vi "Autonomous Independent.vi"   [LabVIEW 2011]
doc: "This VI is called when autonomous begins, and will automatically be terminated when autonomous ends. You can carry out timed or sensor driven robot movement independently without needing to return to the caller."
uses:
  Robot Global Data.vi
  <vilib>/Rock Robotics/WPI/Solenoid/Deprecated/WPI_SolenoidSetBool.vi
types:
  T1 = typedef "WPI_JoystickDevRef.ctl" = cluster{"Device":T2}
  T2 = typedef "WPI_JoystickDeviceEnum.ctl" = enum16{"USB 1", "USB 2", "USB 3", "USB 4", "Kinect 1", "Kinect 2"}
  T3 = cluster{"axis 1 (x)":dbl, "axis 2 (y)":dbl, "axis 3 (throttle)":dbl, "axis 4":dbl, "axis 5":dbl, "axis 6":dbl}
  T4 = enum16{"Tip Bridge", "No Bridge", "Kinect Bridge"}
  T5 = typedef "WPI_SolenoidDevRef.ctl" = cluster{"DevStatus":errorcluster, "Solenoid Module":T6, "Forward Solenoid Channel":T7, "Reverse Solenoid Channel":T7}
  T6 = typedef "FPGA_TypedefSolenoidModule.ctl" = enum16{"Solenoid Module 1", "Solenoid Module 2"}
  T7 = typedef "WPI_SolenoidChannel.ctl" = enum8{"Solenoid 1", "Solenoid 2", "Solenoid 3", "Solenoid 4", "Solenoid 5", "Solenoid 6", "Solenoid 7", "Solenoid 8", "Invalid"}
  T8 = typedef "UDP Dashboard Packet TypeDef.ctl" = cluster{"Distance":dbl, "Shooter Control":cluster{"Manual Enabled":bool, "Manual Distance":dbl, "Power Constant":dbl, "RPM Constant":dbl, "Layup Distance":dbl, "RPM Range":cluster{"Max Percentage":dbl, "Min Percentage":dbl}, "Dt In":dbl}, "Tracking Setpoint":dbl, "Shooter PID gains":cluster{"proportional gain (Kc)":dbl, "integral time (Ti, min)":dbl, "derivative time (Td, min)":dbl}, "Tracking PID gains":cluster{"proportional gain (Kc)":dbl, "integral time (Ti, min)":dbl, "derivative time (Td, min)":dbl}, "Shooter PID gains 2":cluster{"proportional gain (Kc)":dbl, "integral time (Ti, min)":dbl, "derivative time (Td, min)":dbl}, "Tracking Tolerance":dbl, "Tracking Limit":dbl, "Autonomous Ball Collection / Shoot Period":dbl}
  T9 = typedef "WPI_GyroDevRef.ctl" = cluster{"DevStatus":errorcluster, "Analog Module":T10, "Analog Channel":T11, "Offset":dbl, "Gain (VoltsPerDegree/Second)":dbl}
  T10 = typedef "FPGA_TypedefAnalogModule.ctl" = enum16{"Analog Module 1", "Analog Module 2"}
  T11 = typedef "FPGA_AIChannel.ctl" = enum8{"AI 1", "AI 2", "AI 3", "AI 4", "AI 5", "AI 6", "AI 7", "AI 8", "Invalid"}
  T12 = typedef "WPI_RobotDriveDevRef.ctl" = cluster{"DevStatus":errorcluster, "Motors[]":T13[], "Square Inputs":bool, "Max Output":dbl, "Isochronous":bool}
  T13 = typedef "WPI_MotorControlDeviceRef.ctl" = cluster{"DeviceStatus":errorcluster, "Type":enum16{"PWM", "CAN"}, "PWM":cluster{"Digital Module":T14, "PWM Channel":T15, "DeadBand":T16}, "CAN":cluster{"Device Number":u8, "Control Mode":T17, "Semaphore":T18, "Max Vout":dbl}, "Invert":bool, "TransformRef":T19, "InvTransformRef":T19}
  T14 = typedef "FPGA_TypedefDigitalModule.ctl" = enum16{"Digital Module 1", "Digital Module 2"}
  T15 = typedef "FPGA_DIOPWMChannel.ctl" = enum8{"PWM 1", "PWM 2", "PWM 3", "PWM 4", "PWM 5", "PWM 6", "PWM 7", "PWM 8", "PWM 9", "PWM 10", "Invalid"}
  T16 = typedef "WPI_PWMDeadband.ctl" = cluster{"Name":string, "maxPositivePwm":i32, "minPositivePwm":i32, "centerPwm":i32, "maxNegativePwm":i32, "minNegativePwm":i32, "angularRange":u16}
  T17 = typedef "WPI_CANJaguar_ControlMode.ctl" = enum8{"Percent VBus", "Current", "Speed", "Position", "Voltage"}
  T18 = typedef "Semaphore RefNum" = refnum<k1>
  T19 = typedef "WPI_PWMTransform_ConPane.ctl" = refnum<vi>
  T20 = cluster{"Shooter Warmup":bool, "Shooter Allow Fire":bool}
  T21 = typedef "WPI_EncoderDevRef.ctl" = cluster{"DevStatus":errorcluster, "EncoderIndex":T22, "CounterIndex":T23, "DistancePerCount":dbl, "Decoding Type":T24}
  T22 = typedef "FPGA_EncoderIdx.ctl" = enum8{"Enc 0", "Enc 1", "Enc 2", "Enc 3", "Invalid"}
  T23 = typedef "FPGA_CounterCtrSystemIndex.ctl" = enum8{"Ctr 0", "Ctr 1", "Ctr 2", "Ctr 3", "Ctr 4", "Ctr 5", "Ctr 6", "Ctr 7", "Invalid"}
  T24 = typedef "WPI_EncoderType.ctl" = enum16{"1x", "2x", "4x"}
  T25 = typedef "WPI_DigitalInputDevRef.ctl" = cluster{"DevStatus":errorcluster, "DIO Channel":T26, "Digital Module":T14}
  T26 = typedef "FPGA_DIOChannel.ctl" = enum8{"DIO 1", "DIO 2", "DIO 3", "DIO 4", "DIO 5", "DIO 6", "DIO 7", "DIO 8", "DIO 9", "DIO 10", "DIO 11", "DIO 12", "DIO 13", "DIO 14", "Invalid"}
  T27 = typedef "WPI_JoystickButtonState.ctl" = cluster{"Button 1":bool, "Button 2":bool, "Button 3":bool, "Button 4":bool, "Button 5":bool, "Button 6":bool, "Button 7":bool, "Button 8":bool, "Button 9":bool, "Button 10":bool, "Button 11":bool, "Button 12":bool}
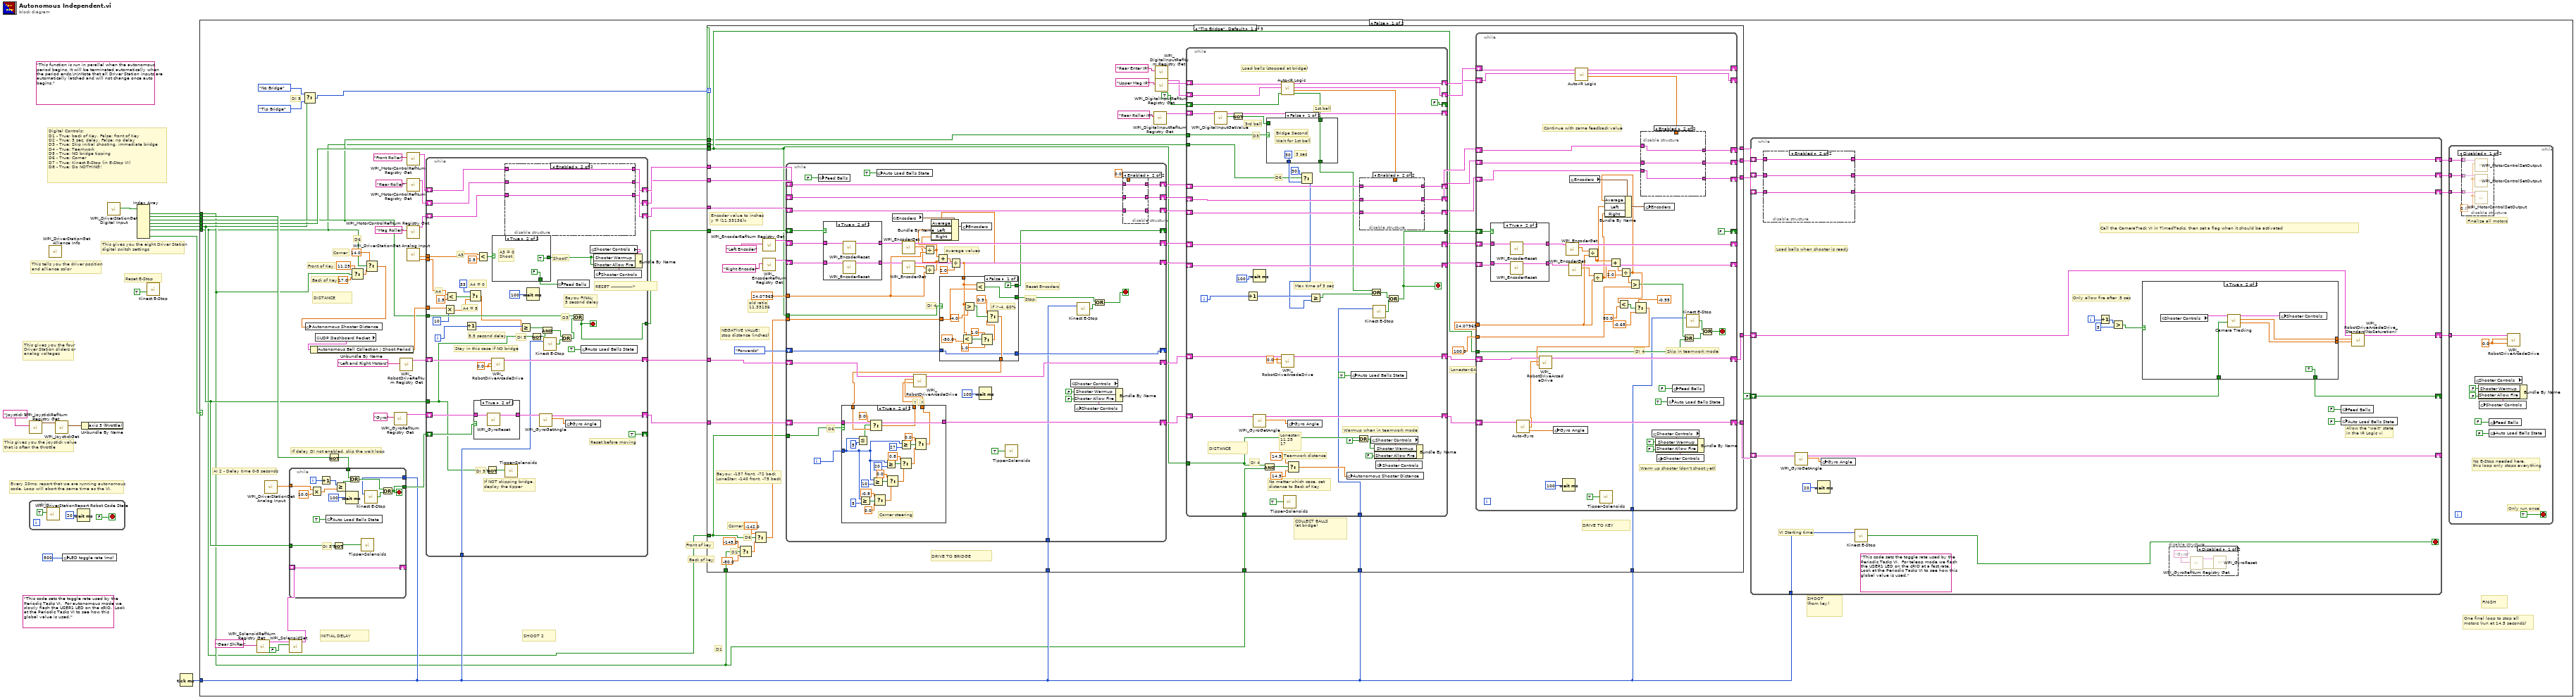
[diagram p0: block diagram]
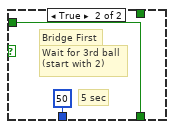
[diagram p3: hidden frame]
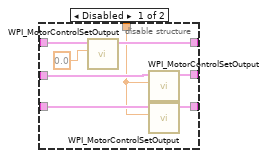
[diagram p4: hidden frame]
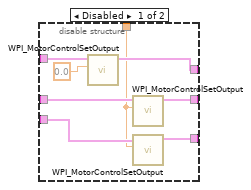
[diagram p5: hidden frame]
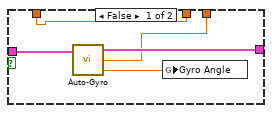
[diagram p7: hidden frame]
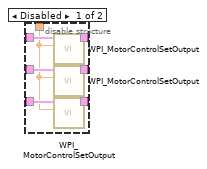
[diagram p8: hidden frame]
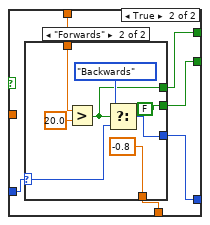
[diagram p9: hidden frame]
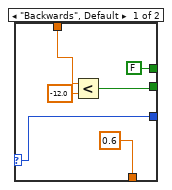
[diagram p10: hidden frame]
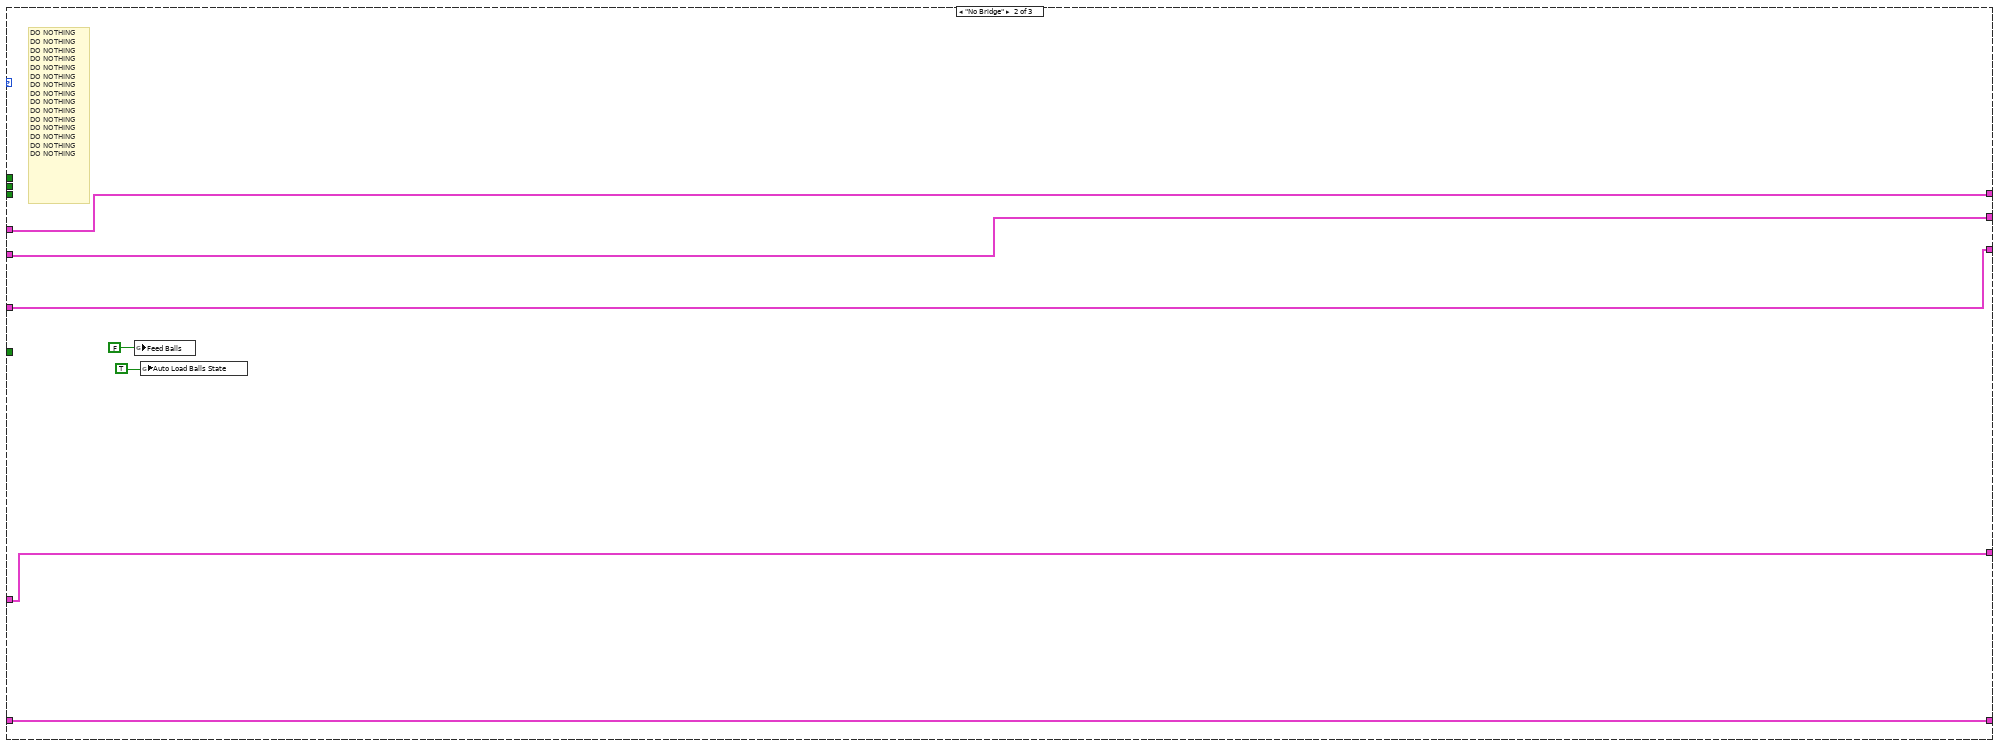
[diagram p12: hidden frame]
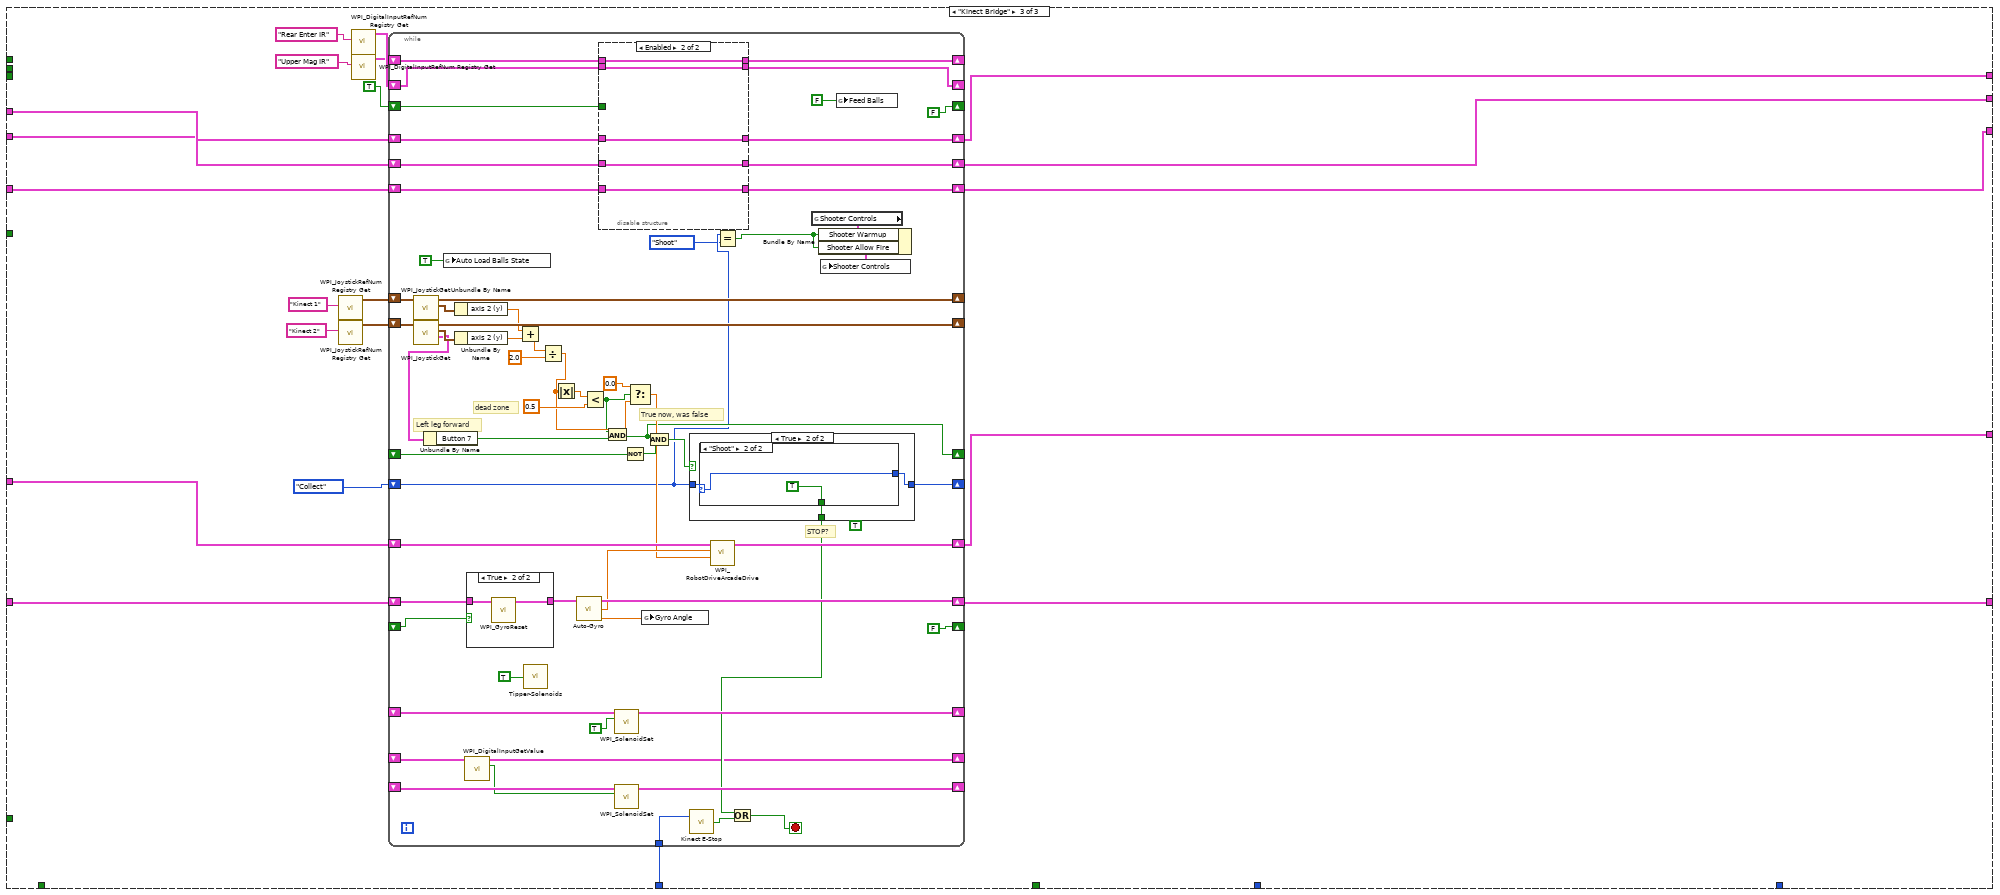
[diagram p13: hidden frame]
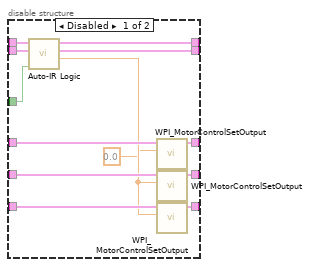
[diagram p14: hidden frame]
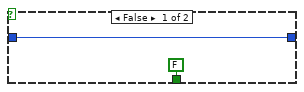
[diagram p15: hidden frame]
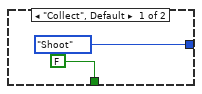
[diagram p16: hidden frame]
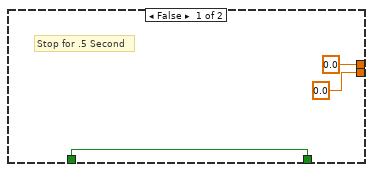
[diagram p18: hidden frame]
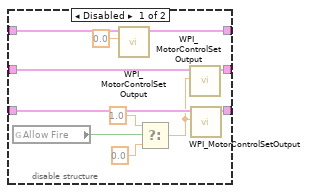
[diagram p20: hidden frame]
diagram:
  (unwired) "This code sets the toggle rate used by the Periodic Tasks VI.  For autonomous mode we slowly flash the USER1 LED on the cRIO.  Look at the Periodic Tasks VI to see how this global value is used."
  (unwired) "This function is run in parallel when the autonomous period begins. It will be terminated automatically when the period ends.\n\nNote that all Driver Station inputs are automatically latched and will not change once auto begins."
  # "Reset E-Stop"
  # "Digital Controls:\nD1 - True: back of Key, False: front of Key\nD2 - True: 3 sec. delay, False: no delay\nD3 - True: Skip initial shooting, immediate bridge\nD4 - True: Teamwork\nD5 - True: NO bridge tipping\nD6 - True: Corner\nD7 - True: Kinect E-Stop (in E-Stop VI)\nD8 - True: Do NOTHING!"
  # "Every 20ms, report that we are running autonomous\ncode. Loop will abort the same time as the VI."
  # "This gives you the joystick value\nthat is often the throttle"
  # "This tells you the driver position\nand alliance color"
  # "This gives you the eight Driver Station\ndigital switch settings"
  # "This gives you the four\nDriver Station sliders or\nanalog voltages"
  n1 = call <vilib>:"WPI_JoystickRefNum Registry Get.vi"("refnum name"="Joystick 1") -> ("JoystickDevRef"=w11:T1)  [unwired: 1 in, 9 out]
  n2 = while {
    stop <- FALSE stop-if-true
    n3 = call <vilib>:"WPI_DriverStationReport Robot Code State.vi"("Autonomous"=TRUE) -> ()  [unwired: 10 in, 1 out]
    n4 = Wait (ms)(milliseconds to wait=u32 20) -> ()  [unwired: 1 out]
  }
  n5 = call <vilib>:"WPI_DriverStationGet Alliance Info.vi"() -> ()  [unwired: 12 out]
  n6 = call <vilib>:"WPI_JoystickGet.vi"("JoystickDevRef"=w11) -> ("Axes"=w12:T3)  [unwired: 1 in, 5 out]
  n7 = global write "Robot Global Data.vi" "LED toggle rate (ms)"(u32 500 ("LED ms toggle rate")) -> ()
  n8 = Unbundle By Name(w12) -> ()  [unwired: 1 out]
  n9 = call <vilib>:"WPI_DriverStationGet Digital Input.vi"() -> ("Driver Station Digital Input (1-8)"=w14:bool[])  [unwired: 11 out]
  n10 = Index Array(array=w14) -> (element #1=w7:bool, element #2=w9:bool, element #3=w1:bool, element #4=w8:bool, element #5=w5:bool, element #6=w2:bool, element #8=w6:bool)  [unwired: 8 in, 1 out]
  n11 = call "Kinect E-Stop.vi"("Reset"=TRUE) -> ()  [unwired: 1 in, 1 out]
  n12 = Tick Count (ms)() -> (millisecond timer value=w4:u32)
  n13 = case shown="False" w6 {
    tunnel: w9 -> [w45 _]
    tunnel: w8 -> [w43 _]
    tunnel: w7 -> [w24 _]
    tunnel: w5 -> [w26 _]
    tunnel: w4 -> [w36 _]
    tunnel: w2 -> [w18 _]
    tunnel: w1 -> [w27 _]
    frame False {
      # "Back of key"
      # "Front of key"
      # "Corner"
      # "D6"
      # "Back of Key"
      # "Front of Key"
      # "RESET --------------->"
      # "FINISH"
      # "SHOOT\n(from key)"
      # "AI 2 - Delay time 0-5 seconds"
      # "SHOOT 2"
      # "INITIAL DELAY"
      # "If delay DI not enabled, skip the wait loop"
      # "One final loop to stop all\nmotors (run at 14.5 seconds)"
      # "DI 5"
      # "DISTANCE"
      # "D1"
      n14 = call <vilib>:"WPI_SolenoidRefNum Registry Get.vi"("refnum name"="Gear Shifter") -> ("SolenoidDevRef"=w34:T5)  [unwired: 9 in, 1 out]
      n15 = call <vilib>:"WPI_DriverStationGet Analog Input.vi"() -> ("Analog 2 (V)"=w44:dbl)  [unwired: 11 out]
      n16 = call-poly <vilib>:"WPI_SolenoidSet.vi"("Value"=FALSE, "SolenoidDevRef"=w34) -> ("SolenoidDevRef"=w33:T5)  [unwired: 8 in, 1 out]
      n17 = Select(t=T4."No Bridge", s=w26, f=T4."Tip Bridge") -> (s? t:f=w25:T4)
      n18 = global read "Robot Global Data.vi" "UDP Dashboard Packet"() -> (w29:T8)
      n19 = Unbundle By Name(w29) -> ("Autonomous Ball Collection / Shoot Period"=w28:dbl)
      n20 = Not(x=w45) -> (.not. x?=w46:bool)
      n21 = while {
        tunnel: [w539] -> w47
        tunnel: w46 -> [w545]
        tunnel: w44 -> [w542]
        shift-right: [w537] -> _
        shift-left: w33 -> [w537]
        tunnel: w36 -> [w538]
        tunnel: w26 -> [w535]
        i -> [w547]
        stop <- w539 stop-if-true
        # "DI 5"
        n22 = Multiply(x=w542, y=10.0) -> (x*y=w544:dbl)
        n23 = Increment(x=w547) -> (x+1=w548:i32)
        n24 = global write "Robot Global Data.vi" "Auto Load Balls State"(TRUE ("Feed Balls")) -> ()
        n25 = Not(x=w535) -> (.not. x?=w536:bool)
        n26 = Greater Or Equal?(x=w548, y=w544) -> (x >= y?=w549:bool)
        n27 = Wait (ms)(milliseconds to wait=u32 100) -> ()  [unwired: 1 out]
        n28 = Or(x=w545, y=w549) -> (x .or. y?=w540:bool)
        n29 = call "Tipper-Solenoids.vi"("Deploy Tipper"=w536) -> ()  [unwired: 1 out]
        n30 = call "Kinect E-Stop.vi"("Start Time"=w538) -> ("Stop"=w541:bool)  [unwired: 1 in]
        n31 = Or(x=w540, y=w541) -> (x .or. y?=w539:bool)
      }
      n32 = Select(t=11.25 ("X axis value"), s=w24, f=17.0 ("X axis value")) -> (s? t:f=w21:dbl)
      n33 = Select(t=14.0 ("X axis value"), s=w18, f=w21) -> (s? t:f=w20:dbl)
      n34 = global write "Robot Global Data.vi" "Autonomous Shooter Distance"(w20) -> ()
      n35 = call <vilib>:"WPI_GyroRefNum Registry Get.vi"("refnum name"="Gyro") -> ("GyroDevRef"=w50:T9)  [unwired: 9 in, 1 out]
      n36 = call <vilib>:"WPI_RobotDriveRefNum Registry Get.vi"("refnum name"="Left and Right Motors") -> ("RobotDriveDevRef"=w59:T12)  [unwired: 9 in, 1 out]
      n37 = call <vilib>:"WPI_MotorControlRefNum Registry Get.vi"("refnum name"="Front Roller") -> ("MotorControlDevRef"=w65:T13)  [unwired: 9 in, 1 out]
      n38 = call <vilib>:"WPI_MotorControlRefNum Registry Get.vi"("refnum name"="Rear Roller") -> ("MotorControlDevRef"=w64:T13)  [unwired: 9 in, 1 out]
      n39 = call <vilib>:"WPI_MotorControlRefNum Registry Get.vi"("refnum name"="Mag Roller") -> ("MotorControlDevRef"=w68:T13)  [unwired: 9 in, 1 out]
      n40 = call <vilib>:"WPI_DriverStationGet Analog Input.vi"() -> ("Analog 4 (V)"=w30:dbl, "Analog 3 (V)"=w31:dbl)  [unwired: 8 in, 2 out]
      n41 = while {
        tunnel: [w621] -> w57
        shift-right: [w639] -> w63
        shift-left: w65 -> [w641]
        shift-right: [w638] -> w62
        shift-left: w64 -> [w640]
        shift-right: [w637] -> w61
        shift-left: w68 -> [w642]
        shift-right: [w634] -> w58
        shift-left: w59 -> [w635]
        shift-right: [w626] -> w49
        shift-left: w50 -> [w631]
        shift-right: [TRUE ("Shooter Enabled")] -> _
        shift-left: w47 -> [w630]
        tunnel: w36 -> [w624]
        tunnel: w26 -> [w600]
        tunnel: w27 -> [w622]
        tunnel: w31 -> [w608]
        tunnel: w30 -> [w606]
        tunnel: w28 -> [w611]
        i -> [w633]
        stop <- w621 stop-if-true
        w636 = 0.0 ("X axis value")
        # "Stay in this case if NO bridge"
        # "DI 5"
        # "A4"
        # "A3"
        # "A4 = 0"
        # "A4 = 5"
        # "Shoot?"
        # "Reset before moving"
        # "D3"
        # "If NOT skipping bridge,\ndeploy the tipper"
        # "DI 5"
        # "Bayou FINAL:\n5 second delay"
        # "5.5 second delay"
        n42 = Multiply(x=w611, y=u32 10) -> (x*y=w612:dbl)
        n43 = Less?(x=w606, y=2.5) -> (x < y?=w605:bool)
        n44 = Increment(x=w633) -> (x+1=w632:i32)
        n45 = Select(t=u32 33 ("y"), s=w605, f=w612) -> (s? t:f=w614:dbl)
        n46 = case shown="True" w630 {
          tunnel: w631 -> [w662 w664]
          tunnel: [w662 w663] -> w627
          frame False {
          }
          frame True {
            n47 = call <vilib>:"WPI_GyroReset.vi"("GyroDevRef"=w664) -> ("GyroDevRef"=w663:T9)  [unwired: 9 in, 1 out]
          }
        }
        n48 = Less?(x=w608, y=2.5) -> (x < y?=w607:bool)
        n49 = Not(x=w600) -> (.not. x?=w623:bool)
        n50 = call-poly <vilib>:"WPI_RobotDriveArcadeDrive.vi"("Y axis value"=w636, "X axis value"=w636, "RobotDriveDevRef"=w635) -> ("RobotDriveDevRef"=w634:T12)  [unwired: 7 in, 1 out]
        n51 = case shown="True" w607 {
          tunnel: [FALSE ("Shooter Enabled") TRUE ("Shooter Enabled")] -> w619
          tunnel: [TRUE ("Shooter Enabled") FALSE ("Shooter Enabled")] -> w616
          frame False {
            # "A3 = 5\nFeed Balls Out"
          }
          frame True {
            # "A3 = 0\nShoot"
          }
        }
        n52 = disable-structure shown="Enabled" {
          disable-tunnel: w642 -> [w658 w659]
          disable-tunnel: w641 -> [w657 w661]
          disable-tunnel: w640 -> [w656 w660]
          disable-tunnel: [w654 w661] -> w639
          disable-tunnel: [w653 w660] -> w638
          disable-tunnel: [w652 w659] -> w637
          frame Disabled {
            # "Load balls when shooter is ready"
            n53 = global read "Robot Global Data.vi" "Allow Fire"() -> (w651:bool)
            n54 = Select(t=1.0 ("Output"), s=w651, f=0.0 ("Output")) -> (s? t:f=w648:dbl)
            n55 = call <vilib>:"WPI_MotorControlSetOutput.vi"("Output"=0.0, "MotorControlDevRef"=w657) -> ("MotorControlDevRef"=w654:T13)  [unwired: 8 in, 1 out]
            n56 = call <vilib>:"WPI_MotorControlSetOutput.vi"("Output"=w648, "MotorControlDevRef"=w656) -> ("MotorControlDevRef"=w653:T13)  [unwired: 8 in, 1 out]
            n57 = call <vilib>:"WPI_MotorControlSetOutput.vi"("Output"=w648, "MotorControlDevRef"=w658) -> ("MotorControlDevRef"=w652:T13)  [unwired: 8 in, 1 out]
          }
          frame Enabled {
          }
        }
        n58 = call "Tipper-Solenoids.vi"("Deploy Tipper"=w623) -> ()  [unwired: 1 out]
        n59 = Greater Or Equal?(x=w632, y=w614) -> (x >= y?=w602:bool)
        n60 = Wait (ms)(milliseconds to wait=u32 100) -> ()  [unwired: 1 out]
        n61 = Not(x=w600) -> (.not. x?=w601:bool)
        n62 = call <vilib>:"WPI_GyroGetAngle.vi"("GyroDevRef"=w627) -> ("Angle"=w628:dbl, "GyroDevRef"=w626:T9)  [unwired: 7 in, 2 out]
        n63 = And(x=w602, y=w601) -> (x .and. y?=w603:bool)
        n64 = call "Kinect E-Stop.vi"("Start Time"=w624) -> ("Stop"=w625:bool)  [unwired: 1 in]
        n65 = global write "Robot Global Data.vi" "Feed Balls"(w616) -> ()
        n66 = Or(x=w603, y=w625) -> (x .or. y?=w620:bool)
        n67 = global write "Robot Global Data.vi" "Gyro Angle"(w628) -> ()
        n68 = Or(x=w622, y=w620) -> (x .or. y?=w621:bool)
        n69 = global write "Robot Global Data.vi" "Auto Load Balls State"(TRUE ("Feed Balls")) -> ()
        n70 = global read "Robot Global Data.vi" "Shooter Controls"() -> (w617:T20)
        n71 = Bundle By Name(cluster=w617, "Shooter Warmup"=w619, "Shooter Allow Fire"=w619) -> (w618:T20)
        n72 = global write "Robot Global Data.vi" "Shooter Controls"(w618) -> ()
      }
      n73 = case shown="\"Tip Bridge\", Default" w25 {
        tunnel: w63 -> [w137 w418 w439]
        tunnel: w62 -> [w136 w417 w438]
        tunnel: w61 -> [w135 w416 w437]
        tunnel: w58 -> [w134 w415 w436]
        tunnel: w57 -> [w133 _ _]
        tunnel: [w131 w415 w419] -> w56
        tunnel: [w130 w418 w423] -> w55
        tunnel: [w129 w417 w422] -> w54
        tunnel: [w128 w416 w421] -> w53
        tunnel: w49 -> [w110 w414 w435]
        tunnel: [w109 w414 w420] -> w48
        tunnel: w43 -> [w105 _ _]
        tunnel: w24 -> [w104 _ _]
        tunnel: w24 -> [w101 _ _]
        tunnel: w36 -> [w96 _ w424]
        tunnel: w36 -> [w95 _ _]
        tunnel: w36 -> [w94 _ _]
        tunnel: w27 -> [w91 _ _]
        tunnel: w18 -> [w87 _ _]
        tunnel: w18 -> [w86 _ _]
        frame "Tip Bridge", Default {
          # "D1"
          # "Corner"
          # "D6"
          # "Lonestar:64"
          # "Bayou: -137 front, -72 back\nLoneStar: -140 front, -75 back"
          # "old ratio\n11.33136"
          # "DRIVE TO KEY"
          # "COLLECT BALLS\n(at bridge)"
          # "DRIVE TO BRIDGE"
          # "NEGATIVE VALUE!\nstop distance (inches)"
          # "Encoder value to inches\ny = (11.33136)x"
          n74 = Select(t=-145.0 ("y"), s=w101, f=-80.0 ("y")) -> (s? t:f=w90:dbl)
          n75 = Select(t=-142.0 ("y"), s=w87, f=w90) -> (s? t:f=w89:dbl)
          n76 = call <vilib>:"WPI_EncoderRefNum Registry Get.vi"("refnum name"="Left Encoder") -> ("EncoderDevRef"=w140:T21)  [unwired: 9 in, 1 out]
          n77 = call <vilib>:"WPI_EncoderRefNum Registry Get.vi"("refnum name"="Right Encoder") -> ("EncoderDevRef"=w139:T21)  [unwired: 9 in, 1 out]
          n78 = while {
            shift-right: [w324] -> w114
            shift-left: w140 -> [w332]
            shift-right: [w328] -> w113
            shift-left: w139 -> [w331]
            tunnel: 24.07965 ("y") -> [w327]
            tunnel: w89 -> [w303]
            shift-right: [w315] -> w118
            shift-left: w134 -> [w319]
            shift-right: [w318] -> w124
            shift-left: w137 -> [w322]
            shift-right: [w317] -> w123
            shift-left: w136 -> [w321]
            shift-right: [w316] -> w122
            shift-left: w135 -> [w320]
            shift-right: [w296] -> w116
            shift-left: w110 -> [w297]
            shift-right: [w302] -> _
            shift-left: w133 -> [w310]
            shift-right: [w304] -> _
            shift-left: enum16{"Backwards", "Forwards"}."Forwards" -> [w305]
            tunnel: w105 -> [w301]
            tunnel: w96 -> [w294]
            tunnel: w87 -> [w286]
            i -> [w285]
            stop <- w298 stop-if-true
            # "Y"
            # "X"
            # "D6"
            # "Stop"
            # "Reset Encoders"
            # "DI 4"
            # "Average values"
            n79 = global write "Robot Global Data.vi" "Feed Balls"(FALSE ("Feed Balls")) -> ()
            n80 = case shown="True" w310 {
              tunnel: w332 -> [w407 w411]
              tunnel: w331 -> [w406 w410]
              tunnel: [w407 w409] -> w329
              tunnel: [w406 w408] -> w330
              frame False {
              }
              frame True {
                n81 = call <vilib>:"WPI_EncoderReset.vi"("EncoderDevRef"=w411) -> ("EncoderDevRef"=w409:T21)  [unwired: 9 in, 1 out]
                n82 = call <vilib>:"WPI_EncoderReset.vi"("EncoderDevRef"=w410) -> ("EncoderDevRef"=w408:T21)  [unwired: 9 in, 1 out]
              }
            }
            n83 = global write "Robot Global Data.vi" "Auto Load Balls State"(TRUE ("Feed Balls")) -> ()
            n84 = global read "Robot Global Data.vi" "Encoders"() -> (w313:cluster{"Average":dbl, "Left":dbl, "Right":dbl})
            n85 = call <vilib>:"WPI_EncoderGet.vi"("EncoderDevRef"=w329) -> ("Distance"=w312:dbl, "EncoderDevRef"=w324:T21)  [unwired: 5 in, 4 out]
            n86 = call <vilib>:"WPI_EncoderGet.vi"("EncoderDevRef"=w330) -> ("Distance"=w311:dbl, "EncoderDevRef"=w328:T21)  [unwired: 5 in, 4 out]
            n87 = Divide(x=w312, y=w327) -> (x/y=w308:dbl)
            n88 = Divide(x=w311, y=w327) -> (x/y=w307:dbl)
            n89 = Add(x=w308, y=w307) -> (x+y=w326:dbl)
            n90 = Divide(x=w326, y=2.0) -> (x/y=w306:dbl)
            n91 = Bundle By Name(cluster=w313, "Average"=w306, "Left"=w308, "Right"=w307) -> (w314:cluster{"Average":dbl, "Left":dbl, "Right":dbl})
            n92 = case shown="False" w301 {
              tunnel: w306 -> [w374 w389]
              tunnel: [w377 w390] -> w284
              tunnel: w305 -> [w376 w391]
              tunnel: [w376 w388] -> w304
              tunnel: w303 -> [w375 _]
              tunnel: [w373 w387] -> w299
              tunnel: [FALSE w386] -> w302
              frame False {
                # "if >-4, 60%"
                n93 = Less?(x=w374, y=-50.0) -> (x < y?=w380:bool)
                n94 = Greater?(x=w374, y=-4.0) -> (0:w384:bool)
                n95 = Less?(x=w374, y=w375) -> (x < y?=w373:bool)
                n96 = Select(t=1.0, s=w380, f=1.0) -> (s? t:f=w381:dbl)
                n97 = Select(t=0.9, s=w384, f=w381) -> (s? t:f=w377:dbl)
              }
              frame True {
                n98 = case shown="\"Forwards\"" w391 {
                  selector: w391 -> [w392 w402]
                  tunnel: [0.6 ("setpoint") -0.8 ("setpoint")] -> w390
                  tunnel: w389 -> [w394 w405]
                  tunnel: [w392 w401] -> w388
                  tunnel: [w396 FALSE] -> w387
                  tunnel: [FALSE w398] -> w386
                  frame "Backwards", Default {
                    n99 = Less?(x=w394, y=-12.0) -> (x < y?=w396:bool)
                  }
                  frame "Forwards" {
                    n100 = Greater?(x=w405, y=20.0) -> (0:w398:bool)
                    n101 = Select(t=enum16{"Backwards", "Forwards"}."Backwards", s=w398, f=w402) -> (s? t:f=w401:enum16{"Backwards", "Forwards"})
                  }
                }
              }
            }
            n102 = case shown="True" w286 {
              tunnel: w297 -> [w337 w361]
              tunnel: [w336 w361] -> w296
              tunnel: [w334 w349] -> w295
              tunnel: w285 -> [_ w339]
              tunnel: w284 -> [w333 w343]
              tunnel: [w333 w342] -> w283
              frame False {
                n103 = call "Auto-Gyro.vi"("GyroDevRef"=w337) -> ("Angle"=w335:dbl, "X-Axis Out"=w334:dbl, "GyroDevRef Out"=w336:T9)  [unwired: 2 in]
                n104 = global write "Robot Global Data.vi" "Gyro Angle"(w335) -> ()
              }
              frame True {
                # "Corner steering"
                n105 = Less Or Equal?(x=w339, y=5) -> (x <= y?=w340:bool)
                n106 = Greater Or Equal?(x=w339, y=5) -> (x >= y?=w347:bool)
                n107 = Select(t=0.0, s=w340, f=w343) -> (s? t:f=w342:dbl)
                n108 = Greater Or Equal?(x=w339, y=10) -> (x >= y?=w359:bool)
                n109 = Select(t=-0.8, s=w347, f=0.0 ("t")) -> (s? t:f=w344:dbl)
                n110 = Greater Or Equal?(x=w339, y=20) -> (x >= y?=w356:bool)
                n111 = Select(t=0.0, s=w359, f=w344) -> (s? t:f=w354:dbl)
                n112 = Select(t=0.8, s=w356, f=w354) -> (s? t:f=w351:dbl)
                n113 = Greater Or Equal?(x=w339, y=27) -> (x >= y?=w350:bool)
                n114 = Select(t=0.0, s=w350, f=w351) -> (s? t:f=w349:dbl)
              }
            }
            n115 = call-poly <vilib>:"WPI_RobotDriveArcadeDrive.vi"("Y axis value"=w283, "X axis value"=w295, "RobotDriveDevRef"=w319) -> ("RobotDriveDevRef"=w315:T12)  [unwired: 7 in, 1 out]
            n116 = global write "Robot Global Data.vi" "Encoders"(w314) -> ()
            n117 = Wait (ms)(milliseconds to wait=u32 100) -> ()  [unwired: 1 out]
            n118 = call "Tipper-Solenoids.vi"("Deploy Tipper"=TRUE) -> ()  [unwired: 1 out]
            n119 = global read "Robot Global Data.vi" "Shooter Controls"() -> (w292:T20)
            n120 = Bundle By Name(cluster=w292, "Shooter Warmup"=FALSE ("Shooter Enabled"), "Shooter Allow Fire"=FALSE ("Shooter Enabled")) -> (w293:T20)
            n121 = global write "Robot Global Data.vi" "Shooter Controls"(w293) -> ()
            n122 = call "Kinect E-Stop.vi"("Start Time"=w294) -> ("Stop"=w300:bool)  [unwired: 1 in]
            n123 = Or(x=w299, y=w300) -> (x .or. y?=w298:bool)
            n124 = disable-structure shown="Enabled" {
              disable-tunnel: w322 -> [w368 w371]
              disable-tunnel: w321 -> [w367 w370]
              disable-tunnel: w320 -> [w366 w369]
              disable-tunnel: [w365 w371] -> w318
              disable-tunnel: [w364 w370] -> w317
              disable-tunnel: [w363 w369] -> w316
              disable-tunnel: 0.0 ("Output") -> [w362 _]
              frame Disabled {
                n125 = call <vilib>:"WPI_MotorControlSetOutput.vi"("Output"=w362, "MotorControlDevRef"=w368) -> ("MotorControlDevRef"=w365:T13)  [unwired: 8 in, 1 out]
                n126 = call <vilib>:"WPI_MotorControlSetOutput.vi"("Output"=w362, "MotorControlDevRef"=w367) -> ("MotorControlDevRef"=w364:T13)  [unwired: 8 in, 1 out]
                n127 = call <vilib>:"WPI_MotorControlSetOutput.vi"("Output"=w362, "MotorControlDevRef"=w366) -> ("MotorControlDevRef"=w363:T13)  [unwired: 8 in, 1 out]
              }
              frame Enabled {
              }
            }
          }
          n128 = call <vilib>:"WPI_DigitalInputRefNum Registry Get.vi"("refnum name"="Rear Roller IR") -> ("DigitalInputDevRef"=w92:T25)  [unwired: 9 in, 1 out]
          n129 = call <vilib>:"WPI_DigitalInputRefNum Registry Get.vi"("refnum name"="Rear Enter IR") -> ("DigitalInputDevRef"=w99:T25)  [unwired: 9 in, 1 out]
          n130 = call <vilib>:"WPI_DigitalInputRefNum Registry Get.vi"("refnum name"="Upper Mag IR") -> ("DigitalInputDevRef"=w98:T25)  [unwired: 9 in, 1 out]
          n131 = while {
            shift-right: [w164] -> w126
            shift-left: w98 -> [w166]
            shift-right: [w165] -> w127
            shift-left: w99 -> [w167]
            tunnel: [w168] -> w125
            shift-right: [w193] -> w121
            shift-left: w124 -> [w194]
            shift-right: [w192] -> w120
            shift-left: w123 -> [w189]
            shift-right: [w191] -> w119
            shift-left: w122 -> [w190]
            shift-right: [w187] -> w117
            shift-left: w118 -> [w188]
            shift-right: [w178] -> w115
            shift-left: w116 -> [w179]
            shift-right: [w184] -> w111
            shift-left: w113 -> [w184]
            shift-right: [w185] -> w112
            shift-left: w114 -> [w185]
            tunnel: w105 -> [w171]
            tunnel: w104 -> [w173]
            shift-right: [FALSE ("Shooter Enabled")] -> _
            shift-left: TRUE ("Shooter Enabled") -> [w162]
            tunnel: w95 -> [w160]
            shift-right: [w153] -> _
            shift-left: w92 -> [w154]
            tunnel: w91 -> [w152]
            tunnel: w86 -> [w143]
            i -> [w181]
            stop <- w168 stop-if-true
            w186 = 0.0 ("X axis value")
            # "D6"
            # "1st ball"
            # "3rd ball"
            # "D3"
            # "Lonestar:\n11.25\n17"
            # "DISTANCE"
            # "No matter which case, set distance to Back of Key"
            # "Teamwork distance"
            # "Warmup when in teamwork mode"
            # "DI 4"
            # "Load balls (stopped at bridge)"
            # "Max time of 3 sec"
            n132 = call <vilib>:"WPI_DigitalInputGetValue.vi"("DigitalInputDevRef"=w154) -> ("Value"=w149:bool, "DigitalInputDevRef"=w153:T25)  [unwired: 8 in, 1 out]
            n133 = Not(x=w149) -> (.not. x?=w148:bool)
            n134 = Increment(x=w181) -> (x+1=w183:i32)
            n135 = Wait (ms)(milliseconds to wait=u32 100) -> ()  [unwired: 1 out]
            n136 = call <vilib>:"WPI_GyroGetAngle.vi"("GyroDevRef"=w179) -> ("Angle"=w180:dbl, "GyroDevRef"=w178:T9)  [unwired: 7 in, 2 out]
            n137 = And(x=w171, y=w173) -> (x .and. y?=w172:bool)
            n138 = call "Auto-IR Logic.vi"("Reset"=w162, "Upper Mag IR"=w166, "Rear Enter IR"=w167) -> ("Finished"=w151:bool, "Roller Output"=w163:dbl, "Upper Mag IR Out"=w164:T25, "Rear Enter IR Out"=w165:T25)  [unwired: 1 in]
            n139 = case shown="False" w152 {
              tunnel: w151 -> [w197 _]
              tunnel: [w197 w199] -> w150
              tunnel: w148 -> [_ w199]
              tunnel: [u32 30 ("y") u32 50 ("y")] -> w146
              frame False {
                # "3 sec"
                # "Wait for 1st ball"
                # "Bridge Second"
              }
              frame True {
                # "5 sec"
                # "Wait for 3rd ball\n(start with 2)"
                # "Bridge First"
              }
            }
            n140 = call-poly <vilib>:"WPI_RobotDriveArcadeDrive.vi"("Y axis value"=w186, "X axis value"=w186, "RobotDriveDevRef"=w188) -> ("RobotDriveDevRef"=w187:T12)  [unwired: 7 in, 1 out]
            n141 = call "Tipper-Solenoids.vi"("Deploy Tipper"=TRUE) -> ()  [unwired: 1 out]
            n142 = Select(t=14.5 ("X axis value"), s=w172, f=14.5 ("X axis value")) -> (s? t:f=w174:dbl)
            n143 = global write "Robot Global Data.vi" "Gyro Angle"(w180) -> ()
            n144 = Select(t=u32 30, s=w143, f=w146) -> (s? t:f=w145:u32)
            n145 = Greater Or Equal?(x=w183, y=w145) -> (x >= y?=w182:bool)
            n146 = global write "Robot Global Data.vi" "Autonomous Shooter Distance"(w174) -> ()
            n147 = global write "Robot Global Data.vi" "Auto Load Balls State"(TRUE ("Feed Balls")) -> ()
            n148 = Or(x=w171, y=FALSE ("Shooter Enabled")) -> (x .or. y?=w156:bool)
            n149 = disable-structure shown="Enabled" {
              disable-tunnel: w194 -> [w207 w210]
              disable-tunnel: [w205 w210] -> w193
              disable-tunnel: [w204 w209] -> w192
              disable-tunnel: [w203 w208] -> w191
              disable-tunnel: w190 -> [w202 w208]
              disable-tunnel: w189 -> [w201 w209]
              disable-tunnel: w163 -> [w200 _]
              frame Disabled {
                n150 = call <vilib>:"WPI_MotorControlSetOutput.vi"("Output"=0.0, "MotorControlDevRef"=w207) -> ("MotorControlDevRef"=w205:T13)  [unwired: 8 in, 1 out]
                n151 = call <vilib>:"WPI_MotorControlSetOutput.vi"("Output"=w200, "MotorControlDevRef"=w201) -> ("MotorControlDevRef"=w204:T13)  [unwired: 8 in, 1 out]
                n152 = call <vilib>:"WPI_MotorControlSetOutput.vi"("Output"=w200, "MotorControlDevRef"=w202) -> ("MotorControlDevRef"=w203:T13)  [unwired: 8 in, 1 out]
              }
              frame Enabled {
              }
            }
            n153 = Or(x=w150, y=w182) -> (x .or. y?=w169:bool)
            n154 = global read "Robot Global Data.vi" "Shooter Controls"() -> (w158:T20)
            n155 = call "Kinect E-Stop.vi"("Start Time"=w160) -> ("Stop"=w170:bool)  [unwired: 1 in]
            n156 = Bundle By Name(cluster=w158, "Shooter Warmup"=w156, "Shooter Allow Fire"=FALSE ("Shooter Enabled")) -> (w159:T20)
            n157 = global write "Robot Global Data.vi" "Shooter Controls"(w159) -> ()
            n158 = Or(x=w169, y=w170) -> (x .or. y?=w168:bool)
          }
          n159 = while {
            shift-right: [w260] -> _
            shift-left: w112 -> [w265]
            shift-right: [w261] -> _
            shift-left: w111 -> [w264]
            tunnel: 24.07965 ("y") -> [w259]
            tunnel: 100.0 ("y") -> [w252]
            shift-right: [w249] -> w131
            shift-left: w117 -> [w251]
            shift-right: [w225] -> w109
            shift-left: w115 -> [w226]
            shift-right: [w245] -> w128
            shift-left: w119 -> [w246]
            shift-right: [w243] -> w130
            shift-left: w121 -> [w244]
            shift-right: [w247] -> w129
            shift-left: w120 -> [w248]
            shift-right: [w220] -> _
            shift-left: w127 -> [w222]
            shift-right: [w219] -> _
            shift-left: w126 -> [w221]
            shift-right: [FALSE] -> _
            shift-left: w125 -> [w242]
            tunnel: w105 -> [w231]
            tunnel: w94 -> [w218]
            stop <- w228 stop-if-true
            # "Skip in teamwork mode"
            # "DI 4"
            # "Continue with same feedback value"
            # "Warm up shooter (don't shoot yet)"
            n160 = case shown="True" w242 {
              tunnel: w265 -> [w278 w282]
              tunnel: w264 -> [w277 w281]
              tunnel: [w278 w280] -> w263
              tunnel: [w277 w279] -> w262
              frame False {
              }
              frame True {
                n161 = call <vilib>:"WPI_EncoderReset.vi"("EncoderDevRef"=w282) -> ("EncoderDevRef"=w280:T21)  [unwired: 9 in, 1 out]
                n162 = call <vilib>:"WPI_EncoderReset.vi"("EncoderDevRef"=w281) -> ("EncoderDevRef"=w279:T21)  [unwired: 9 in, 1 out]
              }
            }
            n163 = call "Auto-Gyro.vi"("GyroDevRef"=w226) -> ("Angle"=w227:dbl, "X-Axis Out"=w224:dbl, "GyroDevRef Out"=w225:T9)  [unwired: 2 in]
            n164 = global write "Robot Global Data.vi" "Gyro Angle"(w227) -> ()
            n165 = Wait (ms)(milliseconds to wait=u32 100) -> ()  [unwired: 1 out]
            n166 = call <vilib>:"WPI_EncoderGet.vi"("EncoderDevRef"=w263) -> ("Distance"=w256:dbl, "EncoderDevRef"=w260:T21)  [unwired: 5 in, 4 out]
            n167 = call <vilib>:"WPI_EncoderGet.vi"("EncoderDevRef"=w262) -> ("Distance"=w255:dbl, "EncoderDevRef"=w261:T21)  [unwired: 5 in, 4 out]
            n168 = global read "Robot Global Data.vi" "Encoders"() -> (w254:cluster{"Average":dbl, "Left":dbl, "Right":dbl})
            n169 = call "Auto-IR Logic.vi"("Upper Mag IR"=w221, "Rear Enter IR"=w222) -> ("Roller Output"=w223:dbl, "Upper Mag IR Out"=w219:T25, "Rear Enter IR Out"=w220:T25)  [unwired: 2 in, 1 out]
            n170 = Divide(x=w256, y=w259) -> (x/y=w240:dbl)
            n171 = Divide(x=w255, y=w259) -> (x/y=w239:dbl)
            n172 = call "Tipper-Solenoids.vi"("Deploy Tipper"=TRUE) -> ()  [unwired: 1 out]
            n173 = Add(x=w240, y=w239) -> (x+y=w258:dbl)
            n174 = Divide(x=w258, y=2.0) -> (x/y=w238:dbl)
            n175 = Bundle By Name(cluster=w254, "Average"=w238, "Left"=w240, "Right"=w239) -> (w253:cluster{"Average":dbl, "Left":dbl, "Right":dbl})
            n176 = Less?(x=w238, y=80.0) -> (x < y?=w236:bool)
            n177 = Greater?(x=w238, y=w252) -> (0:w232:bool)
            n178 = Select(t=-0.95, s=w236, f=-0.65) -> (s? t:f=w233:dbl)
            n179 = call-poly <vilib>:"WPI_RobotDriveArcadeDrive.vi"("Y axis value"=w233, "X axis value"=w224, "RobotDriveDevRef"=w251) -> ("RobotDriveDevRef"=w249:T12)  [unwired: 7 in, 1 out]
            n180 = disable-structure shown="Enabled" {
              disable-tunnel: w248 -> [w273 w275]
              disable-tunnel: [w272 w275] -> w247
              disable-tunnel: w246 -> [w271 w274]
              disable-tunnel: [w270 w274] -> w245
              disable-tunnel: w244 -> [w269 w276]
              disable-tunnel: [w267 w276] -> w243
              disable-tunnel: w223 -> [w266 _]
              frame Disabled {
                n181 = call <vilib>:"WPI_MotorControlSetOutput.vi"("Output"=0.0, "MotorControlDevRef"=w269) -> ("MotorControlDevRef"=w267:T13)  [unwired: 8 in, 1 out]
                n182 = call <vilib>:"WPI_MotorControlSetOutput.vi"("Output"=w266, "MotorControlDevRef"=w273) -> ("MotorControlDevRef"=w272:T13)  [unwired: 8 in, 1 out]
                n183 = call <vilib>:"WPI_MotorControlSetOutput.vi"("Output"=w266, "MotorControlDevRef"=w271) -> ("MotorControlDevRef"=w270:T13)  [unwired: 8 in, 1 out]
              }
              frame Enabled {
              }
            }
            n184 = global write "Robot Global Data.vi" "Encoders"(w253) -> ()
            n185 = global read "Robot Global Data.vi" "Shooter Controls"() -> (w216:T20)
            n186 = Bundle By Name(cluster=w216, "Shooter Warmup"=TRUE ("Shooter Enabled"), "Shooter Allow Fire"=FALSE ("Shooter Enabled")) -> (w217:T20)
            n187 = global write "Robot Global Data.vi" "Shooter Controls"(w217) -> ()
            n188 = global write "Robot Global Data.vi" "Auto Load Balls State"(TRUE ("Feed Balls")) -> ()
            n189 = global write "Robot Global Data.vi" "Feed Balls"(FALSE ("Feed Balls")) -> ()
            n190 = Or(x=w232, y=w231) -> (x .or. y?=w229:bool)
            n191 = call "Kinect E-Stop.vi"("Start Time"=w218) -> ("Stop"=w230:bool)  [unwired: 1 in]
            n192 = Or(x=w230, y=w229) -> (x .or. y?=w228:bool)
          }
        }
        frame "No Bridge" {
          # "DO NOTHING\nDO NOTHING\nDO NOTHING\nDO NOTHING\nDO NOTHING\nDO NOTHING\nDO NOTHING\nDO NOTHING\nDO NOTHING\nDO NOTHING\nDO NOTHING\nDO NOTHING\nDO NOTHING\nDO NOTHING\nDO NOTHING"
          n193 = global write "Robot Global Data.vi" "Feed Balls"(FALSE ("Feed Balls")) -> ()
          n194 = global write "Robot Global Data.vi" "Auto Load Balls State"(TRUE ("Feed Balls")) -> ()
        }
        frame "Kinect Bridge" {
          n195 = call <vilib>:"WPI_JoystickRefNum Registry Get.vi"("refnum name"="Kinect 1") -> ("JoystickDevRef"=w432:T1)  [unwired: 9 in, 1 out]
          n196 = call <vilib>:"WPI_JoystickRefNum Registry Get.vi"("refnum name"="Kinect 2") -> ("JoystickDevRef"=w431:T1)  [unwired: 9 in, 1 out]
          n197 = call <vilib>:"WPI_DigitalInputRefNum Registry Get.vi"("refnum name"="Rear Enter IR") -> ("DigitalInputDevRef"=w427:T25)  [unwired: 9 in, 1 out]
          n198 = call <vilib>:"WPI_DigitalInputRefNum Registry Get.vi"("refnum name"="Upper Mag IR") -> ("DigitalInputDevRef"=w426:T25)  [unwired: 9 in, 1 out]
          n199 = while {
            shift-right: [w496] -> w423
            shift-left: w439 -> [w493]
            shift-right: [w497] -> w422
            shift-left: w438 -> [w494]
            shift-right: [w498] -> w421
            shift-left: w437 -> [w495]
            shift-right: [w485] -> w420
            shift-left: w435 -> [w503]
            shift-right: [w500] -> w419
            shift-left: w436 -> [w499]
            shift-right: [w451] -> _
            shift-left: _ -> [w452]
            shift-right: [w489] -> _
            shift-left: _ -> [w490]
            shift-right: [w487] -> _
            shift-left: _ -> [w488]
            shift-right: [FALSE] -> _
            shift-left: _ -> [w501]
            shift-right: [w478] -> _
            shift-left: w432 -> [w480]
            shift-right: [w477] -> _
            shift-left: w431 -> [w479]
            shift-right: [w462] -> _
            shift-left: _ -> [w463]
            shift-right: [w460] -> _
            shift-left: enum16{"Collect", "Shoot"}."Collect" -> [w445]
            shift-right: [w456] -> _
            shift-left: w427 -> [w458]
            shift-right: [w455] -> _
            shift-left: w426 -> [w457]
            shift-right: [FALSE ("Shooter Enabled")] -> _
            shift-left: TRUE ("Shooter Enabled") -> [w453]
            tunnel: w424 -> [w448]
            stop <- w491 stop-if-true
            (unwired) TRUE ("Shooter Enabled")
            # "STOP?"
            # "True now, was false"
            # "Left leg forward"
            # "dead zone"
            n200 = call <vilib>:"WPI_JoystickGet.vi"("JoystickDevRef"=w480) -> ("Axes"=w476:T3, "JoystickDevRef"=w478:T1)  [unwired: 4 in, 1 out]
            n201 = call <vilib>:"WPI_JoystickGet.vi"("JoystickDevRef"=w479) -> ("Buttons"=w467:T27, "Axes"=w475:T3, "JoystickDevRef"=w477:T1)  [unwired: 4 in]
            n202 = Unbundle By Name(w467) -> ("Button 7"=w465:bool)
            n203 = global write "Robot Global Data.vi" "Auto Load Balls State"(TRUE ("Feed Balls")) -> ()
            n204 = Unbundle By Name(w476) -> ("axis 2 (y)"=w474:dbl)
            n205 = Unbundle By Name(w475) -> ("axis 2 (y)"=w473:dbl)
            n206 = call <vilib>:"WPI_DigitalInputGetValue.vi"("DigitalInputDevRef"=w452) -> ("Value"=w449:bool, "DigitalInputDevRef"=w451:T25)  [unwired: 8 in, 1 out]
            n207 = case shown="True" w501 {
              tunnel: w503 -> [w531 w533]
              tunnel: [w531 w532] -> w486
              frame False {
              }
              frame True {
                n208 = call <vilib>:"WPI_GyroReset.vi"("GyroDevRef"=w533) -> ("GyroDevRef"=w532:T9)  [unwired: 9 in, 1 out]
              }
            }
            n209 = Add(x=w474, y=w473) -> (x+y=w472:dbl)
            n210 = call "Tipper-Solenoids.vi"("Deploy Tipper"=TRUE) -> ()  [unwired: 1 out]
            n211 = Divide(x=w472, y=2.0) -> (x/y=w469:dbl)
            n212 = Absolute Value(x=w469) -> (abs(x)=w482:dbl)
            n213 = call "Auto-Gyro.vi"("GyroDevRef"=w486) -> ("Angle"=w484:dbl, "X-Axis Out"=w483:dbl, "GyroDevRef Out"=w485:T9)  [unwired: 2 in]
            n214 = Less?(x=w482, y=0.5) -> (x < y?=w466:bool)
            n215 = disable-structure shown="Enabled" {
              disable-tunnel: [w516 w517] -> w498
              disable-tunnel: [w515 w518] -> w497
              disable-tunnel: [w514 w519] -> w496
              disable-tunnel: w495 -> [w513 w517]
              disable-tunnel: w494 -> [w512 w518]
              disable-tunnel: w493 -> [w511 w519]
              disable-tunnel: w458 -> [w510 w521]
              disable-tunnel: w457 -> [w509 w520]
              disable-tunnel: [w508 w521] -> w456
              disable-tunnel: [w507 w520] -> w455
              disable-tunnel: w453 -> [w506 _]
              frame Disabled {
                n216 = call "Auto-IR Logic.vi"("Reset"=w506, "Upper Mag IR"=w509, "Rear Enter IR"=w510) -> ("Roller Output"=w505:dbl, "Upper Mag IR Out"=w507:T25, "Rear Enter IR Out"=w508:T25)  [unwired: 1 in, 1 out]
                n217 = call <vilib>:"WPI_MotorControlSetOutput.vi"("Output"=0.0, "MotorControlDevRef"=w511) -> ("MotorControlDevRef"=w514:T13)  [unwired: 8 in, 1 out]
                n218 = call <vilib>:"WPI_MotorControlSetOutput.vi"("Output"=w505, "MotorControlDevRef"=w512) -> ("MotorControlDevRef"=w515:T13)  [unwired: 8 in, 1 out]
                n219 = call <vilib>:"WPI_MotorControlSetOutput.vi"("Output"=w505, "MotorControlDevRef"=w513) -> ("MotorControlDevRef"=w516:T13)  [unwired: 8 in, 1 out]
              }
              frame Enabled {
              }
            }
            n220 = And(x=w466, y=w465) -> (x .and. y?=w462:bool)
            n221 = call-poly <vilib>:"WPI_SolenoidSet.vi"("Value"=TRUE, "SolenoidDevRef"=w490) -> ("SolenoidDevRef"=w489:T5)  [unwired: 8 in, 1 out]
            n222 = call-poly <vilib>:"WPI_SolenoidSet.vi"("Value"=w449, "SolenoidDevRef"=w488) -> ("SolenoidDevRef"=w487:T5)  [unwired: 8 in, 1 out]
            n223 = Not(x=w463) -> (.not. x?=w464:bool)
            n224 = Select(t=0.0, s=w466, f=w469) -> (s? t:f=w468:dbl)
            n225 = global write "Robot Global Data.vi" "Gyro Angle"(w484) -> ()
            n226 = And(x=w462, y=w464) -> (x .and. y?=w461:bool)
            n227 = case shown="True" w461 {
              tunnel: w445 -> [w523 w526]
              tunnel: [w523 w524] -> w460
              tunnel: [FALSE w525] -> w459
              frame False {
              }
              frame True {
                n228 = case shown="\"Shoot\"" w526 {
                  selector: w526 -> [_ w529]
                  tunnel: [FALSE ("Shooter Enabled") TRUE ("Shooter Enabled")] -> w525
                  tunnel: [enum16{"Collect", "Shoot"}."Shoot" w529] -> w524
                  frame "Collect", Default {
                  }
                  frame "Shoot" {
                  }
                }
              }
            }
            n229 = call "Kinect E-Stop.vi"("Start Time"=w448) -> ("Stop"=w492:bool)  [unwired: 1 in]
            n230 = call-poly <vilib>:"WPI_RobotDriveArcadeDrive.vi"("Y axis value"=w468, "X axis value"=w483, "RobotDriveDevRef"=w499) -> ("RobotDriveDevRef"=w500:T12)  [unwired: 7 in, 1 out]
            n231 = Equal?(x=w445, y=enum16{"Collect", "Shoot"}."Shoot") -> (x = y?=w443:bool)
            n232 = Or(x=w459, y=w492) -> (x .or. y?=w491:bool)
            n233 = global read "Robot Global Data.vi" "Shooter Controls"() -> (w446:T20)
            n234 = Bundle By Name(cluster=w446, "Shooter Warmup"=w443, "Shooter Allow Fire"=w443) -> (w447:T20)
            n235 = global write "Robot Global Data.vi" "Shooter Controls"(w447) -> ()
            n236 = global write "Robot Global Data.vi" "Feed Balls"(FALSE ("Feed Balls")) -> ()
          }
        }
      }
      n237 = while {
        shift-right: [w567] -> w41
        shift-left: w53 -> [w570]
        shift-right: [w568] -> w40
        shift-left: w54 -> [w571]
        shift-right: [w569] -> w39
        shift-left: w55 -> [w572]
        shift-right: [w555] -> w42
        shift-left: w56 -> [w556]
        shift-right: [w564] -> _
        shift-left: w48 -> [w565]
        tunnel: w36 -> [w562]
        shift-right: [w552] -> _
        shift-left: FALSE ("Button 3") -> [w560]
        i -> [w561]
        stop <- w563 stop-if-true
        (unwired) "This code sets the toggle rate used by the Periodic Tasks VI.  For teleop mode we flash the USER1 LED on the cRIO at a fast rate.  Look at the Periodic Tasks VI to see how this global value is used."
        # "Allow the \"wait\" state\nin the IR Logic vi"
        # "Call the CameraTrack VI in TimedTasks, then set a flag when it should be activated"
        # "Only allow fire after .5 sec"
        # "VI Starting time"
        # "Load balls when shooter is ready"
        n238 = disable-structure shown="Enabled" {
          disable-tunnel: w572 -> [w596 w599]
          disable-tunnel: w571 -> [w595 w598]
          disable-tunnel: w570 -> [w594 w597]
          disable-tunnel: [w592 w599] -> w569
          disable-tunnel: [w591 w598] -> w568
          disable-tunnel: [w590 w597] -> w567
          frame Disabled {
            n239 = global read "Robot Global Data.vi" "Allow Fire"() -> (w589:bool)
            n240 = call <vilib>:"WPI_MotorControlSetOutput.vi"("Output"=0.0, "MotorControlDevRef"=w596) -> ("MotorControlDevRef"=w592:T13)  [unwired: 8 in, 1 out]
            n241 = Select(t=1.0 ("Output"), s=w589, f=0.0 ("Output")) -> (s? t:f=w586:dbl)
            n242 = call <vilib>:"WPI_MotorControlSetOutput.vi"("Output"=w586, "MotorControlDevRef"=w595) -> ("MotorControlDevRef"=w591:T13)  [unwired: 8 in, 1 out]
            n243 = call <vilib>:"WPI_MotorControlSetOutput.vi"("Output"=w586, "MotorControlDevRef"=w594) -> ("MotorControlDevRef"=w590:T13)  [unwired: 8 in, 1 out]
          }
          frame Enabled {
          }
        }
        n244 = call <vilib>:"WPI_GyroGetAngle.vi"("GyroDevRef"=w565) -> ("Angle"=w566:dbl, "GyroDevRef"=w564:T9)  [unwired: 7 in, 2 out]
        n245 = Wait (ms)(milliseconds to wait=u32 20) -> ()  [unwired: 1 out]
        n246 = global write "Robot Global Data.vi" "Gyro Angle"(w566) -> ()
        n247 = call "Kinect E-Stop.vi"("Start Time"=w562) -> ("Stop"=w563:bool)  [unwired: 1 in]
        n248 = Increment(x=w561) -> (x+1=w559:i32)
        n249 = Greater?(x=w559, y=5) -> (0:w557:bool)
        n250 = case shown="True" w557 {
          tunnel: w560 -> [w574 w580]
          tunnel: [0.0 ("Drive X") w579] -> w554
          tunnel: [0.0 ("Drive Y") w578] -> w553
          tunnel: [w574 TRUE ("Button 3")] -> w552
          frame False {
            # "Stop for .5 Second"
          }
          frame True {
            n251 = global read "Robot Global Data.vi" "Shooter Controls"() -> (w582:T20)
            n252 = call "Camera Tracking.vi"("Was Tracking"=w580, "Shooter Controls"=w582) -> ("Drive Y"=w578:dbl, "Drive X"=w579:dbl, "Shooter Controls Out"=w581:T20)  [unwired: 5 in, 2 out]
            n253 = global write "Robot Global Data.vi" "Shooter Controls"(w581) -> ()
          }
        }
        n254 = disable-structure shown="Disabled" {
          frame Disabled {
            n255 = call <vilib>:"WPI_GyroRefNum Registry Get.vi"("refnum name"="Gyro") -> ("error out"=w585:errorcluster, "GyroDevRef"=w584:T9)  [unwired: 9 in]
            n256 = call <vilib>:"WPI_GyroReset.vi"("error in (no error)"=w585, "GyroDevRef"=w584) -> ()  [unwired: 8 in, 2 out]
          }
          frame Enabled {
          }
        }
        n257 = global write "Robot Global Data.vi" "Feed Balls"(FALSE ("Feed Balls")) -> ()
        n258 = global write "Robot Global Data.vi" "Auto Load Balls State"(FALSE ("Feed Balls")) -> ()
        n259 = call <vilib>:"WPI_RobotDriveArcadeDrive_Standard(NoSaturation).vi"("Y axis value"=w553, "X axis value"=w554, "RobotDriveDevRef"=w556) -> ("RobotDriveDevRef"=w555:T12)  [unwired: 1 in, 7 out]
      }
      n260 = while {
        tunnel: w42 -> [w79]
        tunnel: w41 -> [w76]
        tunnel: w40 -> [w77]
        tunnel: w39 -> [w78]
        stop <- TRUE stop-if-true
        w80 = 0.0 ("Y axis value")
        # "No E-Stop needed here,\nthis loop only stops everything"
        # "Finalize all motors"
        # "Only run once"
        n261 = disable-structure shown="Disabled" {
          disable-tunnel: w78 -> [w85 _]
          disable-tunnel: w77 -> [w84 _]
          disable-tunnel: w76 -> [w83 _]
          frame Disabled {
            w82 = 0.0 ("Output")
            n262 = call <vilib>:"WPI_MotorControlSetOutput.vi"("Output"=w82, "MotorControlDevRef"=w85) -> ()  [unwired: 8 in, 2 out]
            n263 = call <vilib>:"WPI_MotorControlSetOutput.vi"("Output"=w82, "MotorControlDevRef"=w84) -> ()  [unwired: 8 in, 2 out]
            n264 = call <vilib>:"WPI_MotorControlSetOutput.vi"("Output"=w82, "MotorControlDevRef"=w83) -> ()  [unwired: 8 in, 2 out]
          }
          frame Enabled {
          }
        }
        n265 = global read "Robot Global Data.vi" "Shooter Controls"() -> (w74:T20)
        n266 = Bundle By Name(cluster=w74, "Shooter Warmup"=FALSE ("Shooter Enabled"), "Shooter Allow Fire"=FALSE ("Shooter Enabled")) -> (w75:T20)
        n267 = global write "Robot Global Data.vi" "Shooter Controls"(w75) -> ()
        n268 = global write "Robot Global Data.vi" "Feed Balls"(FALSE ("Camera Track")) -> ()
        n269 = global write "Robot Global Data.vi" "Auto Load Balls State"(FALSE ("Feed Balls")) -> ()
        n270 = call-poly <vilib>:"WPI_RobotDriveArcadeDrive.vi"("Y axis value"=w80, "X axis value"=w80, "RobotDriveDevRef"=w79) -> ()  [unwired: 7 in, 2 out]
      }
    }
    frame True {
      # "DO NOTHING!!!!!!\nDO NOTHING!!!!!!\nDO NOTHING!!!!!!\nDO NOTHING!!!!!!\nDO NOTHING!!!!!!\nDO NOTHING!!!!!!\nDO NOTHING!!!!!!\nDO NOTHING!!!!!!\nDO NOTHING!!!!!!\nDO NOTHING!!!!!!\nDO NOTHING!!!!!!\nDO NOTHING!!!!!!\nDO NOTHING!!!!!!\nDO NOTHING!!!!!!\nDO NOTHING!!!!!!\nDO NOTHING!!!!!!\nDO NOTHING!!!!!!\nDO NOTHING!!!!!!\nDO NOTHING!!!!!!\nDO NOTHING!!!!!!\nDO NOTHING!!!!!!\nDO NOTHING!!!!!!\nDO NOTHING!!!!!!\nDO NOTHING!!!!!!\nDO NOTHING!!!!!!\nDO NOTHING!!!!!!\nDO NOTHING!!!!!!\nDO NOTHING!!!!!!\nDO NOTHING!!!!!!\nDO NOTHING!!!!!!\nDO NOTHING!!!!!!\nDO NOTHING!!!!!!\nDO NOTHING!!!!!!\nDO NOTHING!!!!!!\nDO NOTHING!!!!!!\nDO NOTHING!!!!!!\nDO NOTHING!!!!!!\nDO NOTHING!!!!!!\nDO NOTHING!!!!!!\nDO NOTHING!!!!!!\nDO NOTHING!!!!!!\nDO NOTHING!!!!!!\nDO NOTHING!!!!!!\nDO NOTHING!!!!!!\nDO NOTHING!!!!!!\nDO NOTHING!!!!!!\nDO NOTHING!!!!!!\nDO NOTHING!!!!!!\nDO NOTHING!!!!!!\nDO NOTHING!!!!!!\nDO NOTHING!!!!!!\nDO NOTHING!!!!!!\nDO NOTHING!!!!!!\nDO NOTHING!!!!!!\nDO NOTHING!!!!!!\nDO NOTHING!!!!!!"
    }
  }
